vi "channel tofromstring.vi"() -> ()   [LabVIEW 2013, in "TBM Tests.lvlib"]
uses:
  TBM Tests.lvlib
  channel/TBM channel.lvclass
panel:
  out "ok?":bool
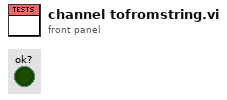
[diagram p1: front panel]
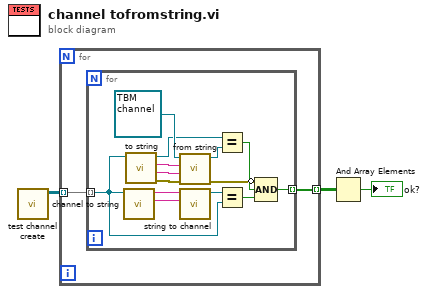
[diagram p0: block diagram]
diagram:
  n1 = call "test channel create.vi"() -> ("chans"=w3:refnum<class "TBM channel.lvclass">[][])  [unwired: 8 in, 3 out]
  n2 = for {
    tunnel: w3 -> [w5] mode=indexing
    tunnel: [w4] -> w2 mode=indexing
    n3 = for {
      tunnel: w5 -> [w14] mode=indexing
      tunnel: [w15] -> w4 mode=indexing
      n4 = call "channel to string.vi"("channel in"=w14) -> ("channel data"=w18:string, "identifier"=w19:string)  [unwired: 9 in]
      n5 = call-dynamic "to string.vi"("channel in"=w14) -> ("error out"=w6:errorcluster, "channel data"=w11:string, "identifier"=w12:string, "channel out"=w9:refnum<class "TBM channel.lvclass">)  [unwired: 7 in]
      n6 = call-dynamic "from string.vi"("error in"=w6, "channel data"=w11, "identifier"=w12, "channel in"=refnum<class "TBM channel.lvclass"> refnum) -> ("error out"=w7:errorcluster, "channel out"=w10:refnum<class "TBM channel.lvclass">)  [unwired: 6 in]
      n7 = call "string to channel.vi"("channel data"=w18, "identifier"=w19) -> ("channel in"=w17:refnum<class "TBM channel.lvclass">)  [unwired: 9 in]
      n8 = Equal?(x=w9, y=w10) -> (x = y?=w8:bool)
      n9 = Equal?(x=w17, y=w14) -> (x = y?=w16:bool)
      n10 = Compound Arithmetic op=AND(invert w7, w8, w16) -> (w15:bool)
    }
  }
  n11 = And Array Elements(Boolean array=w2) -> (logical AND=→"ok?":bool)
